vi "Dashboard Main.vi"() -> ()   [LabVIEW 2012]
uses:
  <vilib>/Utility/sysdir.llb/System Directory Type.ctl
  <vilib>/event_ctls.llb/eventvkey.ctl
  <vilib>/Utility/config.llb/Read Key (String).vi
  <vilib>/Utility/config.llb/Read Key (I32).vi
  <vilib>/Utility/config.llb/Write Key (String).vi
  <vilib>/Utility/config.llb/Write Key (I32).vi
  <vilib>/Utility/config.llb/NI_LVConfig.lvlib
panel:
  out "PitchMin":dbl
  out "PitchMax":dbl
  in  "Auto Align OFF":bool
  in  "Auto Pitch OFF":bool
  in  "Enabled Overlay":T1
  out "Status":T2(ring)
  out "Pitch MotorSlide":dbl(slide) scale=-1.0..1.0 scale format="%#_2e"
  out "Pitch MotorChart":dbl(graph)
  out "Shooter MotorSlide":dbl(slide) scale=-1.0..1.0 scale format="%#_2e"
  out "Shooter MotorChart":dbl(graph)
  out "Battery Value":dbl(slide) scale=0.0..14.0 scale format="%#_2e"
  out "Battery":sgl(graph)
  out "Robot IP":string
  out "JS1 Z":dbl(slide) scale=-1.0..1.0 scale format="%#_2e"
  out "JS2 Z":dbl(slide) scale=-1.0..1.0 scale format="%#_2e"
  out "Joystick 1":cluster{"X":dbl, "Y":dbl}[](graph)
  out "Joystick 2":cluster{"X":dbl, "Y":dbl}[](graph)
  out "JS Buttons 1":T3
  out "JS Buttons 2":T3
  out "MotorSlide4":dbl(slide) scale=-1.0..1.0 scale format="%#_2e"
  out "MotorChart4":dbl(graph)
  out "MotorSlide3":dbl(slide) scale=-1.0..1.0 scale format="%#_2e"
  out "MotorSlide2":dbl(slide) scale=-1.0..1.0 scale format="%#_2e"
  out "MotorChart3":dbl(graph)
  out "MotorChart2":dbl(graph)
  out "MotorSlide1":dbl(slide) scale=-1.0..1.0 scale format="%#_2e"
  out "MotorChart1":dbl(graph)
  out "Buttons 1":cluster{"1":bool, "2":bool, "3":bool}
  out "Kinect 1":cluster{"X":dbl, "Y":dbl, "Z":dbl} {"X" scale=1.0..-1.0; "Y" scale=1.0..-1.0; "Z" scale=1.0..-1.0}
  out "Buttons 2":cluster{"1":bool, "2":bool, "3":bool}
  out "Kinect 2":cluster{"X":dbl, "Y":dbl, "Z":dbl} {"X" scale=1.0..-1.0; "Y" scale=1.0..-1.0; "Z" scale=1.0..-1.0}
  out "Version":string
  out "Skeleton Picture":picture
  out "Players":i8
  out "Image Error":errorcluster
  in  "Camera Settings":T4={"Frate Rate"=15, "Compression"=49, "Size"=1} {"Frate Rate" scale=1.0..30.0; "Size" items=["640x480", "320x240", "160x120"]}
  out "Camera IP":string
  in  "Dashboard Tab":T5(tab)
  in  "Mark PitchF":bool
  in  "Current Pitch":dbl
  in  "Pitch Firing":dbl
  in  "Pitch Loading":dbl
  in  "AutoTargetPitch":dbl
  out "Invert Drive":bool
  out "Fine Control Mode":bool
  out "KickerOut":dbl
  out "Angel Eye":bool
  out "Auto Align":bool
  in  "AutoTargetRotation":dbl
  out "Mode":T6(ring)=enum."Auto Disabled"
  out "# of records":i64
  in  "Mark":bool
  out "Distance":string
  out "Full Array":dbl[][](array[numeric])
  out "SelectedGoalSubarray":dbl[](array[numeric])
  in  "Slider":dbl(slide) scale=0.0..100.0 scale format="%#_3g"
  in  "On/Off":bool caption="Solenoid"
  in  "Test Name":u16(ring) items=["Select the test to run...", "Example Test", "-------------------------------", "List of tests is built in robot code.", "Replace with your own automated tests."]
  in  "Test Tree":string(tree)
  in  "Motor":cluster{"Value":dbl, "Enable":bool} {"Value" scale=-1.0..1.0 scale format="%#_3g"}
  out "Progress":T7 {"Test Progress" scale=0.0..100.0}
  in  "Rev/Fwd":cluster{"Forward":bool, "Reverse":bool}
  in  "Ring":u16(ring) items=["Auto", "Fixed indoor", "Fixed outdoor 1", "Fixed outdoor 2", "Fixed fluorescent 1", "Fixed fluorescent 2", "Hold current"]
  in  "Listbox":i32(listbox)
  in  "Viewer":enum32{"Camera Image", "Variables"}(tab)
  out "Mbps":dbl format="%#.1g"
  in  "Enable":bool
  in  "DB Camera Config":bool
  out "Mbps":bool
  out "fps":dbl format="%#.1g"
  out "Image Error Message":string="Timeout in Camera Communications"
  out "Camera Image":T8(plugin-control)
  out "Tree":string(tree)
  out "Boolean 7":bool
  out "Boolean 6":bool
  out "Boolean 5":bool
  out "Boolean 4":bool
  out "Boolean 3":bool
  out "Boolean 2":bool
  out "Boolean":bool
  # "Drive & Motors"
  # "Rear Left"
  # "Rear Right"
  # "Front Left"
  # "Front Right"
  # "Shooter"
  # "Pitch Control"
  # "Robot IP:"
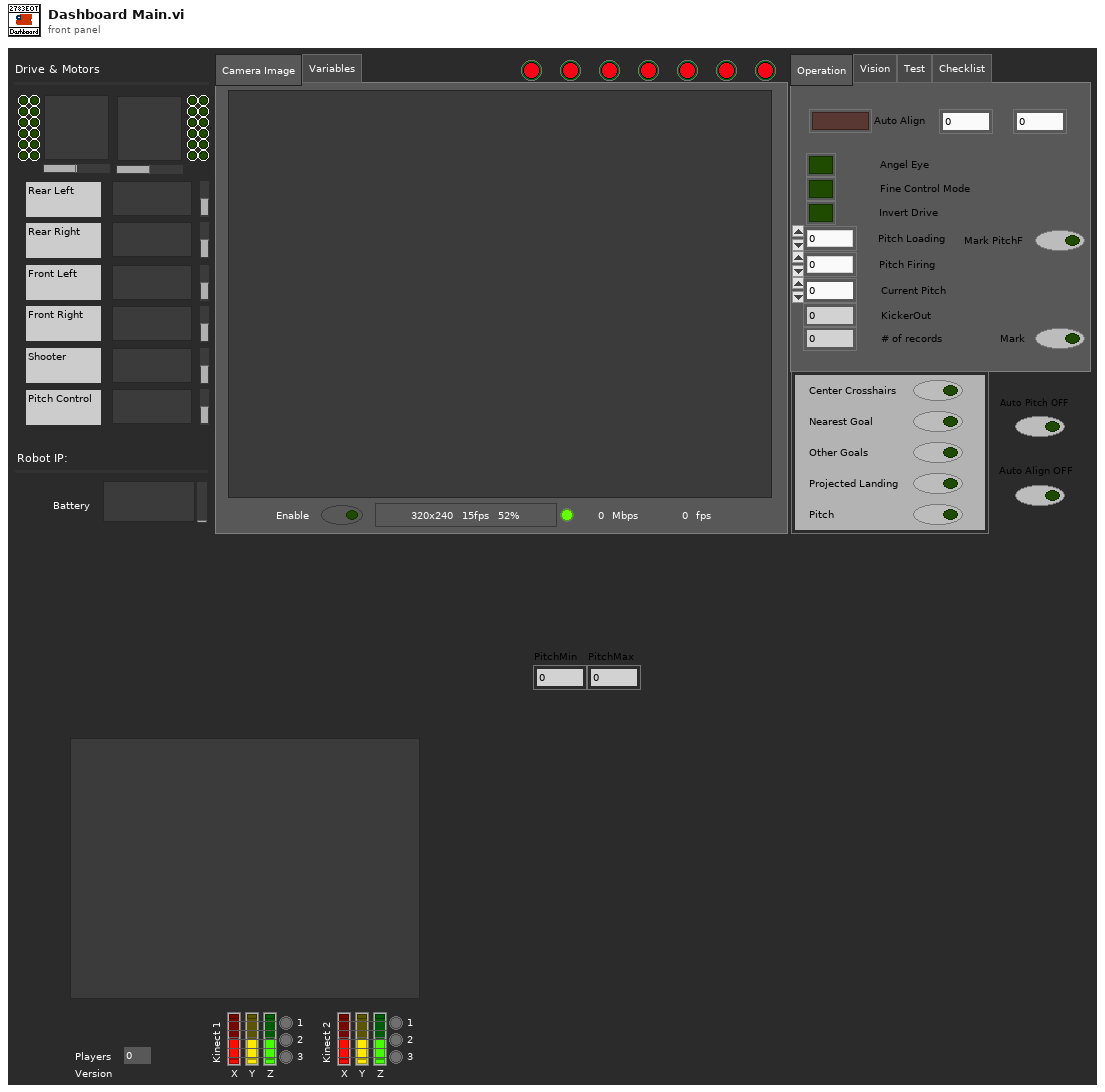
[diagram p1: front panel]
types:
  T1 = cluster{"Center Crosshairs":bool, "Nearest Goal":bool, "Other Goals":bool, "Projected Landing":bool, "Pitch":bool}
  T2 = enum8{"Disconnected", "E-Stop", "Disabled", "Enabled"}
  T3 = cluster{bool, bool, bool, bool, bool, bool, bool, bool, bool, bool, bool, bool}
  T4 = cluster{"Frate Rate":i32, "Compression":i32, "Size":u16}
  T5 = enum32{"Operation", "Vision", "Test", "Checklist"}
  T6 = enum8{"Tele-Op Disabled", "Tele-Op Enabled", "Auto Disabled", "Auto Enabled", "Test Disabled", "Test Enabled", ""}
  T7 = cluster{"Test Progress":u8, "Test Progress Text":string}
  T8 = typedef "IMAQ Image.ctl" = refnum<image>
  T9 = cluster{"Time":string, "Step":string, "Description":string}
  T10 = enum16{"open", "replace", "create", "open or create", "replace or create", "replace or create with confirmation"}
  T11 = cluster{"Joystick 1":cluster{"X":dbl, "Y":dbl}[], "JS Buttons 1":cluster{bool, bool, bool, bool, bool, bool, bool, bool, bool, bool, bool, bool}, "Joystick 2":cluster{"X":dbl, "Y":dbl}[], "JS Buttons 2":cluster{bool, bool, bool, bool, bool, bool, bool, bool, bool, bool, bool, bool}, "AutoTargetRotation":dbl, "AutoTargetPitch":dbl, "Fine Control Mode":bool, "Auto Align":bool, "Current Pitch":dbl, "Full Array":dbl[][], "SelectedGoalSubarray":dbl[], "Distance":string}
  T12 = typedef "System Directory Type.ctl" = i32
  T13 = typedef "Image Type" = u32
  T14 = typedef "AviRefnum.ctl" = refnum<k1>
  T15 = typedef "LVBoundsTypeDef.ctl" = cluster{"Width":u32, "Height":u32}
  T16 = typedef "SkeletonTrackState.ctl" = enum32{"NotTracked", "PositionOnly", "Tracked"}
  T17 = cluster{"TrackingState":u8[], "Position":cluster{"x":sgl, "y":sgl, "z":sgl}, cluster{"x":sgl, "y":sgl, "z":sgl, sgl}[], "TrackState":T16}
  T18 = cluster{cluster{"ScaledToPercentRange":dbl, "ScaledToPercentRange":dbl, "ScaledToPercentRange":dbl}, cluster{bool, bool, bool}}[]
  T19 = cluster{cluster{"ScaledToPercentRange":dbl, "ScaledToPercentRange":dbl, "ScaledToPercentRange":dbl}, cluster{bool, bool, bool}}
  T20 = cluster{"ScaledToPercentRange":dbl, "ScaledToPercentRange":dbl, "ScaledToPercentRange":dbl}
  T21 = typedef "LVRectTypeDef.ctl" = cluster{"Left":i16, "Top":i16, "Right":i16, "Bottom":i16}
  T22 = cluster{"PitchMin":dbl, "PitchMax":dbl, "Pitch Firing":dbl, "Pitch Loading":dbl, "Current Pitch":dbl}
  T23 = cluster{"Competition mode":bool, "Robot Link":bool, "Autonomous":bool, "Enabled":bool, "E-Stop":bool, "Simulated":bool, "TestMode":bool, "Docked Window":bool}
  T24 = cluster{"Boolean Array[0]":bool, "Boolean Array[1]":bool, "Boolean Array[2]":bool, "Boolean Array[3]":bool, "Boolean Array[4]":bool, "Boolean Array[5]":bool, "Boolean Array[6]":bool, "Boolean Array[7]":bool, "Boolean Array[8]":bool, "Boolean Array[9]":bool, "Boolean Array[10]":bool, "Boolean Array[11]":bool}
  T25 = typedef "NI_LVConfig.lvlib/Config Data RefNum.ctl" = refnum<k1>
  T26 = typedef "eventvkey.ctl" = enum16{"ASCII", "Enter", "Return", "Shift", "Ctrl", "Alt", "Cmd", "Opt", "Caps", "NumLock", "Clear", "Break", "Up", "Down", "Left", "Right", "Insert", "Delete", "Home", "End", "PageUp", "PageDown", "Escape", "Help", "Pause", "ScrollLock", "F1", "F2", "F3", "F4", "F5", "F6", "F7", "F8", "F9", "F10", "F11", "F12", "F13", "F14", "F15", "F16", "F17", "F18", "F19", "F20", "F21", "F22", "F23", "F24", "Play", "VolumeUp", "VolumeDown", "Mute", "Two Byte Char"}
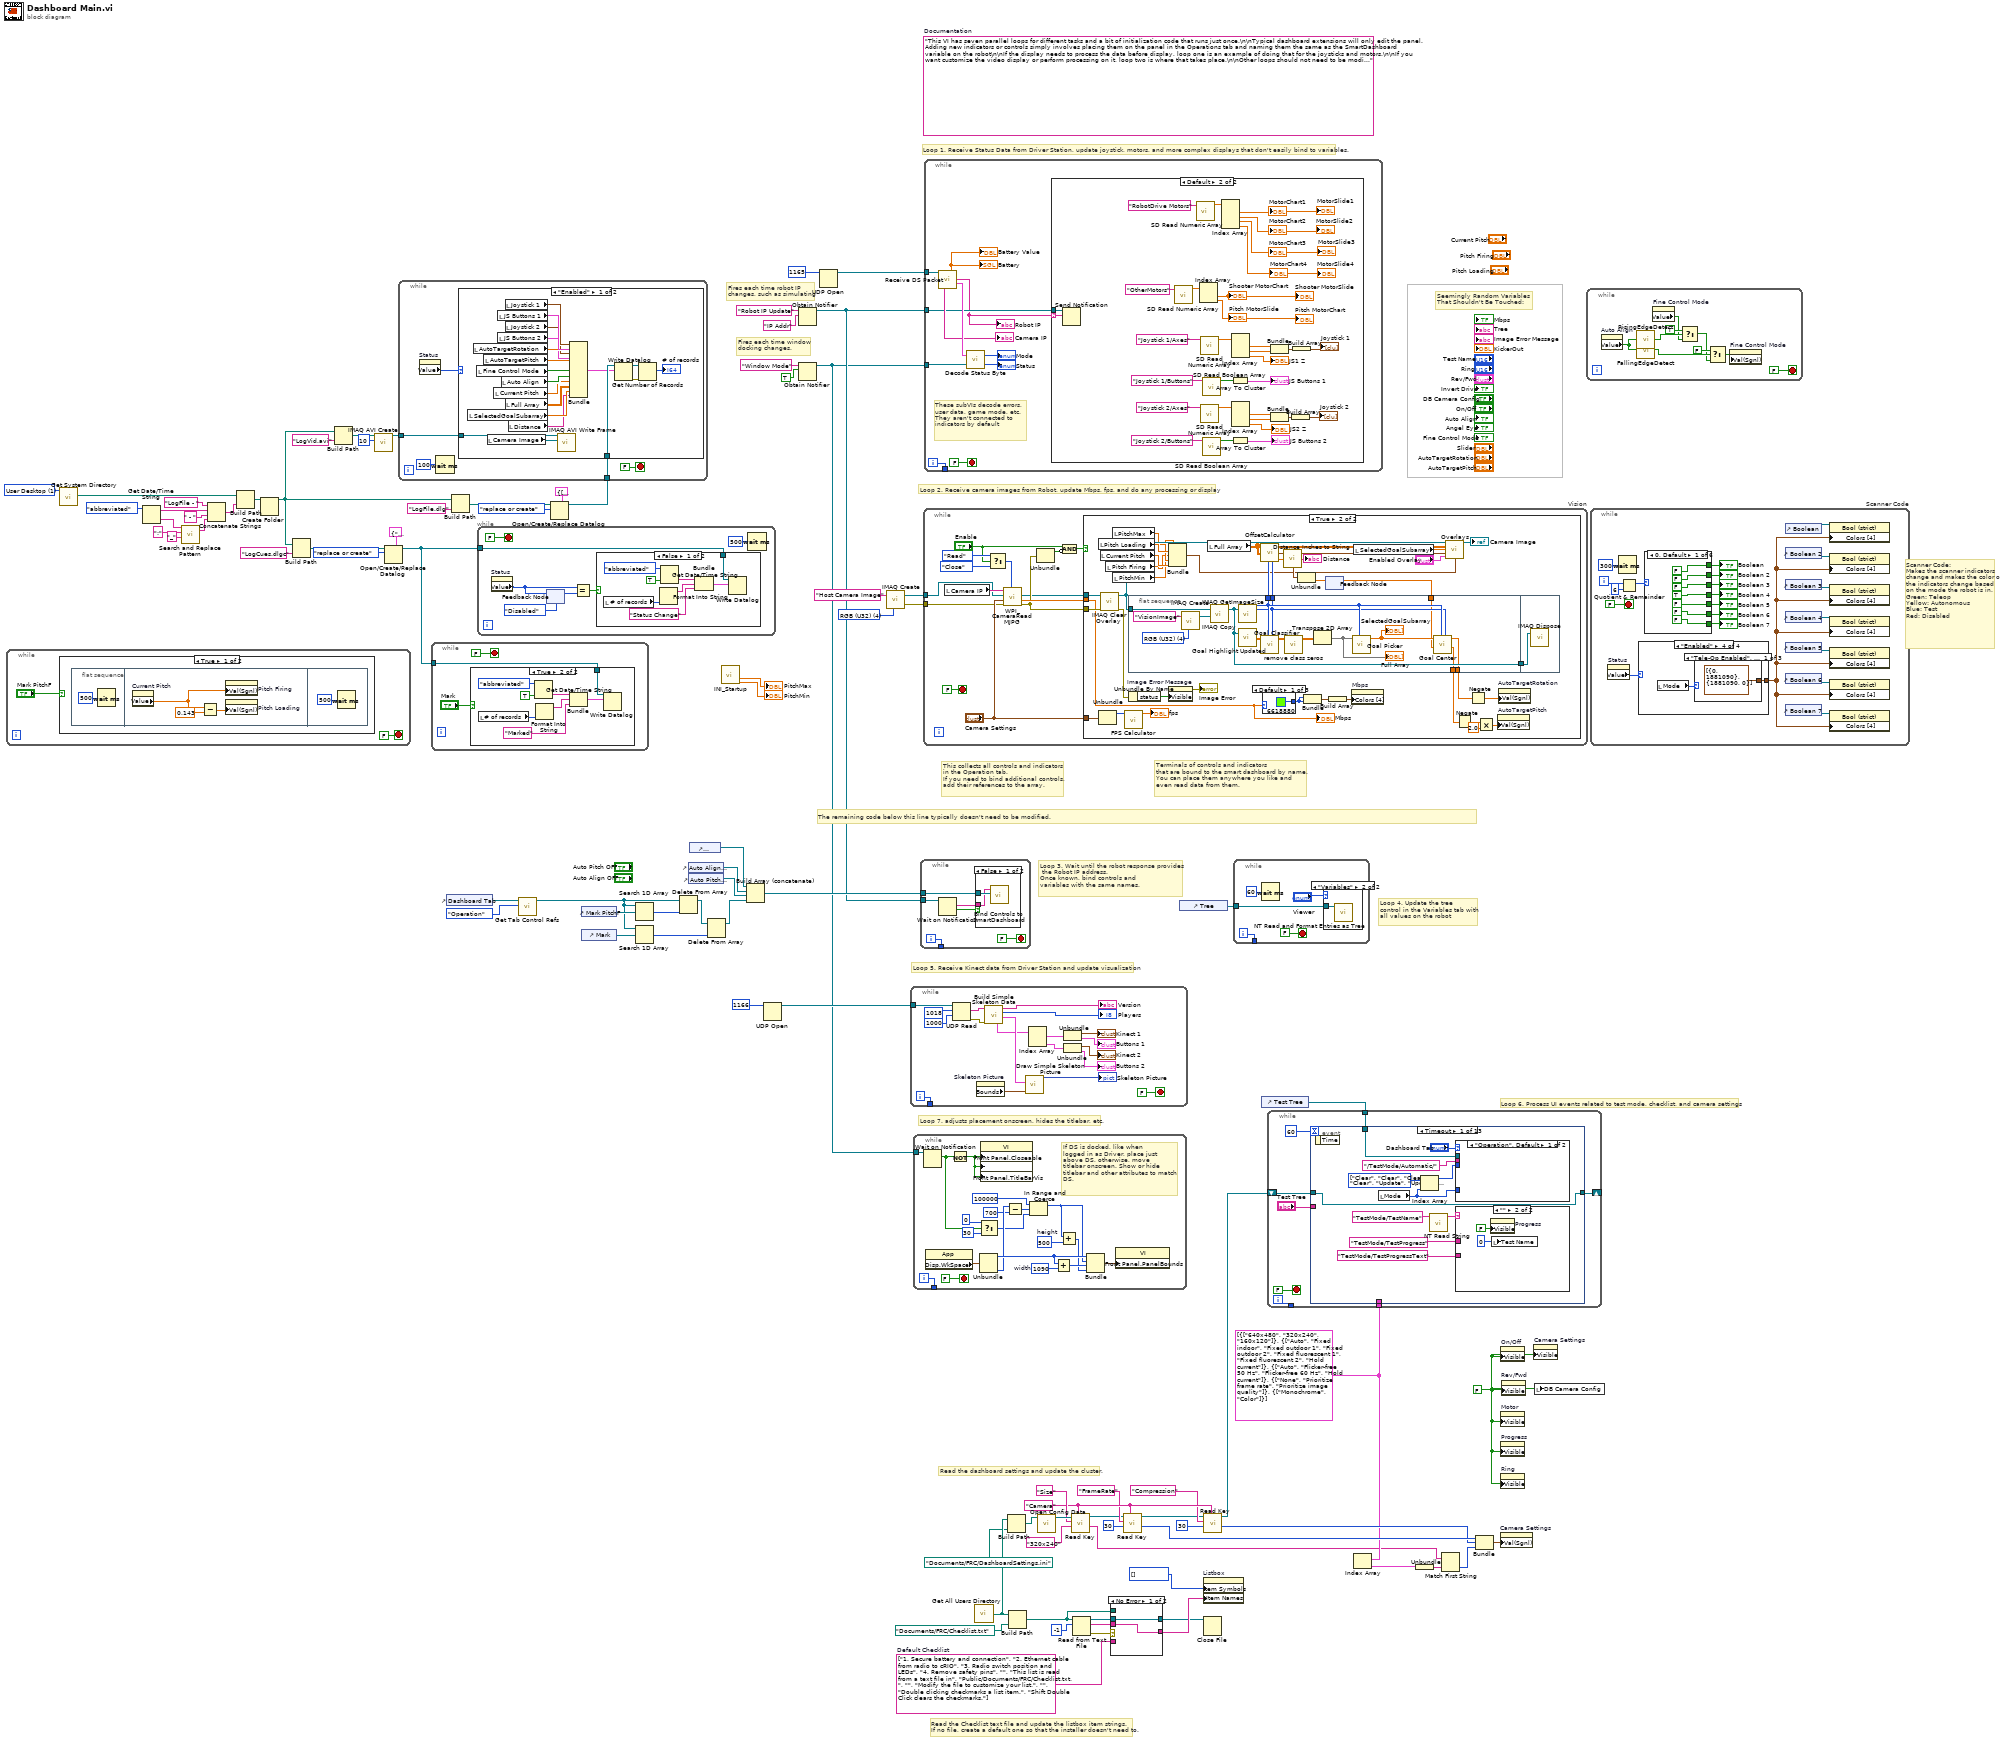
[diagram p0: block diagram]
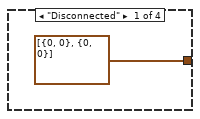
[diagram p6: hidden frame]
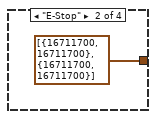
[diagram p7: hidden frame]
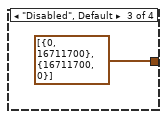
[diagram p8: hidden frame]
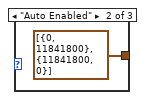
[diagram p9: hidden frame]
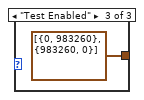
[diagram p10: hidden frame]
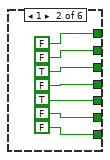
[diagram p11: hidden frame]
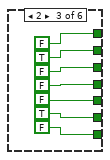
[diagram p12: hidden frame]
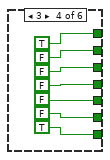
[diagram p13: hidden frame]
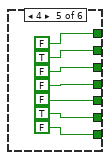
[diagram p14: hidden frame]
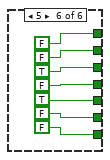
[diagram p15: hidden frame]
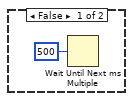
[diagram p17: hidden frame]
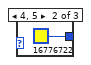
[diagram p18: hidden frame]
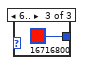
[diagram p19: hidden frame]
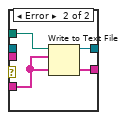
[diagram p20: hidden frame]
diagram:
  w36 = T12 1 items=["User Home"=0, "User Desktop"=1, "User Documents"=2, "User Application Data"=3, "User Preferences"=4, "User Temporary"=5, "Public Documents"=6, "Public Application Data"=7, "Public Preferences"=8, "Public Cache"=13, "System Core Libraries"=9, "System Installed Libraries"=10, "Application Files"=11, "Boot Volume Root"=12] ("system directory type")
  w62 = "Camera"
  w54 = cluster{string[]}[] [{["640x480", "320x240", "160x120"]}, {["Auto", "Fixed indoor", "Fixed outdoor 1", "Fixed outdoor 2", "Fixed fluorescent 1", "Fixed fluorescent 2", "Hold current"]}, {["Auto", "Flicker-free 50 Hz", "Flicker-free 60 Hz", "Hold current"]}, {["None", "Prioritize frame rate", "Prioritize image quality"]}, {["Monochrome", "Color"]}]
  w70 = string[] ["1. Secure battery and connection", "2. Ethernet cable from radio to cRIO", "3. Radio switch position and LEDs", "4. Remove safety pins", "", "This list is read from a text file in", "Public/Documents/FRC/Checklist.txt.", "", "Modify the file to customize your list.", "", "Double clicking checkmarks a list item.", "Shift Double Click clears the checkmarks."]  # Default Checklist
  w68 = FALSE ("Visible")
  (unwired) "This VI has seven parallel loops for different tasks and a bit of initialization code that runs just once.\n\nTypical dashboard extensions will only edit the panel. Adding new indicators or controls simply involves placing them on the panel in the Operations tab and naming them the same as the SmartDashboard variable on the robot\n\nIf the display needs to process the data before display, loop one is an example of doing that for the joysticks and motors.\n\nIf you want customize the video display or perform processing on it, loop two is where that takes place.\n\nOther loops should not need to be modified. They are pretty standard, and document the task they perform."  # Documentation
  w88 = T13 4 items=["Grayscale (U8)", "Grayscale (I16)", "Grayscale (SGL)", "Complex (CSG)", "RGB (U32)", "HSL (U32)", "RGB (U64)"] ("Image Type")
  # "Scanner Code:\nMakes the scanner indicators change and makes the color of the indicators change based on the mode the robot is in.\nGreen: Teleop\nYellow: Autonomous\nBlue: Test\nRed: Disabled"
  # "Seemingly Random Variables That Shouldn't Be Touched:"
  # "Fires each time robot IP\nchanges, such as simulating"
  # "Fires each time window\ndocking changes."
  # "Read the Checklist text file and update the listbox item strings.\nIf no file, create a default one so that the installer doesn't need to."
  # "This collects all controls and indicators\nin the Operation tab.\nIf you need to bind additional controls,\nadd their references to the array."
  # "The remaining code below this line typically doesn't need to be modified."
  # "Loop 6. Process UI events related to test mode, checklist, and camera settings"
  # "Read the dashboard settings and update the cluster."
  # "Terminals of controls and indicators\nthat are bound to the smart dashboard by name.\nYou can place them anywhere you like and\neven read data from them."
  # "Loop 4. Update the tree\ncontrol in the Variables tab with\nall values on the robot"
  # "Loop 3. Wait until the robot response provides\n the Robot IP address.\nOnce known, bind controls and\nvariables with the same names."
  # "Loop 5. Receive Kinect data from Driver Station and update visualization"
  # "Loop 7. adjusts placement onscreen, hides the titlebar, etc."
  # "Loop 1. Receive Status Data from Driver Station, update joystick, motors, and more complex displays that don't easily bind to variables."
  # "Loop 2. Receive camera images from Robot, update Mbps, fps, and do any processing or display"
  n1 = while {
    stop <- FALSE stop-if-true
    n2 = case shown="True" "Mark PitchF" {
      frame True {
        n3 = flat-sequence {
          frame #0 {
            n4 = Wait (ms)(milliseconds to wait=u32 500) -> ()  [unwired: 1 out]
          }
          frame #1 {
            n5 = property on="Current Pitch" class="DigNum (strict)"() -> ("Value"=w96:dbl)  [unwired: 2 in, 2 out]
            n6 = Subtract(x=w96, y=0.143) -> (x-y=w97:dbl)
            n7 = property on="Pitch Firing" class="DigNum (strict)"("Val(Sgnl)"=w96) -> ()  [unwired: 2 in, 2 out]
            n8 = property on="Pitch Loading" class="DigNum (strict)"("Val(Sgnl)"=w97) -> ()  [unwired: 2 in, 2 out]
          }
          frame #2 {
            n9 = Wait (ms)(milliseconds to wait=u32 500) -> ()  [unwired: 1 out]
          }
        }
      }
      frame False {
      }
    }
  }
  n10 = call <vilib>:"Get System Directory.vi"("system directory type"=w36) -> ("system directory"=w25:path)  [unwired: 10 in]
  n11 = Get Date/Time String(date format (0)=enum16{"short", "long", "abbreviated"}."abbreviated") -> (date string=w23:string, time string=w17:string)  [unwired: 2 in]
  n12 = call <vilib>:"Search and Replace Pattern.vi"("string"=w17, "regular expression (\"\")"=":" ("search string/char (-)"), "replace string (\"\")"="_" ("replace string (\"\")")) -> ("result string"=w20:string)  [unwired: 2 in, 1 out]
  n13 = Concatenate Strings("LogFile - " ("string"), w23, " - " ("string"), w20) -> (w21:string)
  n14 = Build Path(base path=w25, name or relative path=w21) -> (appended path=w27:path)
  n15 = Create Folder(path (use dialog)=w27) -> (created path=w12:path)  [unwired: 2 in, 2 out]
  n16 = Build Path(base path=w12, name or relative path="LogCues.dlgc") -> (appended path=w10:path)
  n17 = Build Path(base path=w12, name or relative path="LogVid.avi") -> (appended path=w29:path)
  n18 = call "IMAQ AVI Create"("Frames Per Second"=u32 10, "AVI Path"=w29) -> ("Avi Refnum"=w28:T14)  [unwired: 8 in, 1 out]
  n19 = Open/Create/Replace Datalog(5:T9 {"Time"="", "Step"="", "Description"=""}, 10:T10."replace or create" ("operation (0:open)"), 11:w10) -> (3:w8:refnum<k1>)  [unwired: 3 in, 2 out]
  n20 = while {
    tunnel: w8 -> [w100]
    stop <- FALSE stop-if-true
    n21 = case shown="True" "Mark" {
      tunnel: w100 -> [_ w105]
      frame False {
      }
      frame True {
        n22 = local read "# of records"() -> (w102:i64)
        n23 = Get Date/Time String(date format (0)=enum16{"short", "long", "abbreviated"}."abbreviated", want seconds? (F)=TRUE) -> (time string=w109:string)  [unwired: 1 in, 1 out]
        n24 = Format Into String(w102) -> (resulting string=w103:string)  [unwired: 3 in, 1 out]
        n25 = Bundle("time string"=w109, w103, "Marked") -> (w104:cluster{"time string":string, string, string})  [unwired: 1 in]
        n26 = Write Datalog(6:w104, 7:w105) -> ()  [unwired: 1 in, 2 out]
      }
    }
  }
  n27 = control-ref of="Dashboard Tab"() -> (w84:refnum<vi>)
  n28 = Build Path(base path=w12, name or relative path="LogFile.dlg") -> (appended path=w35:path)
  n29 = while {
    tunnel: w8 -> [w114]
    stop <- FALSE stop-if-true
    n30 = property on="Status" class="Enum (strict)"() -> ("Value"=w111:T2)  [unwired: 2 in, 2 out]
    n31 = feedback-in #1(w111) -> ()
    n32 = feedback #1(T2."Disabled" ("Status")) -> (w112:T2)
    n33 = Equal?(x=w111, y=w112) -> (x = y?=w115:bool)
    n34 = case shown="False" w115 {
      tunnel: w114 -> [w119 _]
      frame False {
        n35 = local read "# of records"() -> (w117:i64)
        n36 = Format Into String(w117) -> (resulting string=w118:string)  [unwired: 3 in, 1 out]
        n37 = Get Date/Time String(date format (0)=enum16{"short", "long", "abbreviated"}."abbreviated", want seconds? (F)=TRUE) -> (time string=w124:string)  [unwired: 1 in, 1 out]
        n38 = Bundle("time string"=w124, w118, "Status Change") -> (w120:cluster{"time string":string, string, string})  [unwired: 1 in]
        n39 = Write Datalog(6:w120, 7:w119) -> ()  [unwired: 1 in, 2 out]
      }
      frame True {
      }
    }
    n40 = Wait (ms)(milliseconds to wait=u32 500) -> ()  [unwired: 1 out]
  }
  n41 = call <vilib>:"Get Tab Control Refs.vi"("Page Index"=enum32{"Operation", "Test"}."Operation" ("Dashboard Tab"), "TabControl in"=w84) -> ("ControlsOnPage"=w1:refnum<vi>[])  [unwired: 9 in]
  n42 = Open/Create/Replace Datalog(5:T11 {"Joystick 1"=[], "JS Buttons 1"={FALSE, FALSE, FALSE, FALSE, FALSE, FALSE, FALSE, FALSE, FALSE, FALSE, FALSE, FALSE}, "Joystick 2"=[], "JS Buttons 2"={FALSE, FALSE, FALSE, FALSE, FALSE, FALSE, FALSE, FALSE, FALSE, FALSE, FALSE, FALSE}, "AutoTargetRotation"=0.0, "AutoTargetPitch"=0.0, "Fine Control Mode"=FALSE, "Auto Align"=FALSE, "Current Pitch"=0.0, "Full Array"=[], "SelectedGoalSubarray"=[], "Distance"=""} ("output cluster"), 10:T10."replace or create" ("operation (0:open)"), 11:w35) -> (3:w33:refnum<k1>)  [unwired: 3 in, 2 out]
  n43 = while {
    tunnel: w33 -> [w129]
    tunnel: w28 -> [w126]
    stop <- FALSE stop-if-true
    n44 = property on="Status" class="Enum (strict)"() -> ("Value"=w125:T2)  [unwired: 2 in, 2 out]
    n45 = Wait (ms)(milliseconds to wait=u32 100) -> ()  [unwired: 1 out]
    n46 = case shown="\"Enabled\"" w125 {
      tunnel: w129 -> [w148 _]
      tunnel: w126 -> [w133 _]
      frame "Enabled" {
        n47 = local read "SelectedGoalSubarray"() -> (w137:dbl[])
        n48 = local read "AutoTargetRotation"() -> (w143:dbl)
        n49 = local read "Fine Control Mode"() -> (w141:bool)
        n50 = local read "AutoTargetPitch"() -> (w142:dbl)
        n51 = local read "Camera Image"() -> (w134:T8)
        n52 = local read "Current Pitch"() -> (w139:dbl)
        n53 = local read "JS Buttons 1"() -> (w146:T3)
        n54 = local read "JS Buttons 2"() -> (w144:T3)
        n55 = local read "Auto Align"() -> (w140:bool)
        n56 = local read "Joystick 1"() -> (w147:cluster{"X":dbl, "Y":dbl}[])
        n57 = local read "Joystick 2"() -> (w145:cluster{"X":dbl, "Y":dbl}[])
        n58 = local read "Full Array"() -> (w138:dbl[][])
        n59 = local read "Distance"() -> (w135:string)
        n60 = call "IMAQ AVI Write Frame"("Image"=w134, "Avi Refnum"=w133) -> ()  [unwired: 8 in, 2 out]
        n61 = Bundle("Joystick 1"=w147, "JS Buttons 1"=w146, "Joystick 2"=w145, "JS Buttons 2"=w144, "AutoTargetRotation"=w143, "AutoTargetPitch"=w142, "Fine Control Mode"=w141, "Auto Align"=w140, "Current Pitch"=w139, "Full Array"=w138, "SelectedGoalSubarray"=w137, "Distance"=w135) -> (w136:T11)  [unwired: 1 in]
        n62 = Write Datalog(6:w136, 7:w148) -> (0:w131:errorcluster, 3:w132:refnum<k1>)  [unwired: 1 in]
        n63 = Get Number of Records(4:w131, 7:w132) -> (2:→"# of records":i64)  [unwired: 2 out]
      }
      frame "Disabled", Default {
      }
    }
  }
  n64 = control-ref of="Mark PitchF"() -> (w6:refnum<vi>)
  n65 = control-ref of="Mark"() -> (w7:refnum<vi>)
  n66 = Search 1D Array(1D array=w1, element=w6) -> (index of element=w5:i32)  [unwired: 1 in]
  n67 = Search 1D Array(1D array=w1, element=w7) -> (index of element=w4:i32)  [unwired: 1 in]
  n68 = Delete From Array(array=w1, index=w5) -> (array with subset deleted=w3:refnum<vi>[])  [unwired: 1 in, 1 out]
  n69 = control-ref of="Auto Align OFF"() -> (w39:refnum<vi>)
  n70 = control-ref of="Auto Pitch OFF"() -> (w38:refnum<vi>)
  n71 = control-ref of="AutoTargetPitch"() -> (w37:refnum<vi>)
  n72 = Delete From Array(array=w3, index=w4) -> (array with subset deleted=w2:refnum<vi>[])  [unwired: 1 in, 1 out]
  n73 = call "INI_Startup.vi"() -> ("PitchMin"=→"PitchMin":dbl, "PitchMax"=→"PitchMax":dbl)  [unwired: 4 in, 2 out]
  n74 = Build Array (concatenate)(w37, w39, w38, w2) -> (w91:refnum<vi>[])
  n75 = UDP Open(11:u16 1166 ("port")) -> (port=w85:refnum<k16>)  [unwired: 2 in, 4 out]
  n76 = Obtain Notifier(name (unnamed)="Robot IP Update", notification data type="IP Addr" ("name (unnamed)")) -> (notifier out=w81:refnum<notifier>)  [unwired: 2 in, 2 out]
  n77 = Obtain Notifier(name (unnamed)="Window Mode", notification data type=TRUE) -> (notifier out=w74:refnum<notifier>)  [unwired: 2 in, 2 out]
  n78 = UDP Open(11:u16 1165 ("port")) -> (port=w89:refnum<k16>)  [unwired: 2 in, 4 out]
  n79 = call "IMAQ Create"("Image Name"="Host Camera Image", "Image Type"=w88) -> ("New Image"=w41:T8, "error out"=w40:errorcluster)  [unwired: 2 in, 1 out]
  n80 = while {
    tunnel: w85 -> [w165]
    tunnel: [w150] -> _
    i -> [w150]
    stop <- FALSE stop-if-true
    n81 = UDP Read(connection ID=w165, max size (548)=1018 ("bytes to read"), timeout ms (25000)=1000) -> (data out=w159:string, error out=w149:errorcluster)  [unwired: 1 in, 3 out]
    n82 = property on="Skeleton Picture" class="Pict"() -> ("Bounds"=w161:T15)  [unwired: 2 in, 2 out]
    n83 = call "Build Simple Skeleton Data.vi"("error in (no error)"=w149, "data in"=w159) -> ("Skeleton Data"=w160:T17, "NumPlayers"=→"Players":i8, "Version String"=→"Version":string, "Simple Joystick Info"=w157:T18)  [unwired: 5 in, 1 out]
    n84 = call "Draw Simple Skeleton Picture.vi"("Bounds"=w161, "Simple Skeleton"=w160) -> ("new picture out"=→"Skeleton Picture":picture)  [unwired: 9 in]
    n85 = Index Array(array=w157) -> (element #1=w156:T19, element #2=w155:T19)  [unwired: 2 in]
    n86 = Unbundle(w156) -> (→"Kinect 1":T20, →"Buttons 1":cluster{bool, bool, bool})
    n87 = Unbundle(w155) -> (→"Kinect 2":T20, →"Buttons 2":cluster{bool, bool, bool})
  }
  n88 = while {
    tunnel: w74 -> [w186]
    tunnel: [w185] -> _
    i -> [w185]
    stop <- FALSE stop-if-true
    w177 = 1090  # width
    w180 = 500  # height
    # "If DS is docked, like when\nlogged in as Driver, place just\nabove DS, otherwise, move\ntitlebar onscreen. Show or hide\ntitlebar and other attributes to match\nDS."
    n89 = Wait on Notification(notifier=w186) -> (notification=w172:bool)  [unwired: 3 in, 3 out]
    n90 = property class="App"() -> ("Disp.WkSpace"=w183:T21)  [unwired: 2 in, 2 out]
    n91 = Not(x=w172) -> (.not. x?=w168:bool)
    n92 = Unbundle(w183) -> ("Left"=w181:i16, "Bottom"=w178:i16)  [unwired: 2 out]
    n93 = Select(t=0, s=w172, f=30) -> (s? t:f=w171:i32)
    n94 = property class="VI"("Front Panel.Closeable"=w168, "Front Panel.Minimizeable"=w168, "Front Panel.TitleBarVis"=w168) -> ()  [unwired: 2 in, 2 out]
    n95 = Subtract(x=w178, y=700) -> (x-y=w175:i32)
    n96 = In Range and Coerce(upper limit=100000, x=w175, lower limit=w171) -> (coerced(x)=w169:i32)  [unwired: 1 out]
    n97 = Add(x=w181, y=w177) -> (x+y=w182:i32)
    n98 = Add(x=w169, y=w180) -> (x+y=w179:i32)
    n99 = Bundle("Left"=w181, w169, w182, w179) -> (w184:cluster{"Left":i16, i32, i32, i32})  [unwired: 1 out]
    n100 = property class="VI"("Front Panel.PanelBounds"=w184) -> ()  [unwired: 2 in, 2 out]
  }
  n101 = while {
    tunnel: w91 -> [w193]
    tunnel: w81 -> [w190]
    tunnel: [w188] -> _
    i -> [w188]
    stop <- FALSE stop-if-true
    n102 = Wait on Notification(notifier=w190) -> (notification=w189:string, timed out?=w191:bool)  [unwired: 3 in, 2 out]
    n103 = case shown="False" w191 {
      tunnel: w193 -> [w195 _]
      tunnel: w189 -> [w194 _]
      frame False {
        n104 = call <vilib>:"Bind Controls to SmartDashboard.vi"("Bound Control Refs"=w195, "Server IP Address"=w194) -> ()  [unwired: 10 in]
      }
      frame True {
      }
    }
  }
  n105 = while "Vision" {
    tunnel: w40 -> [w199]
    tunnel: w41 -> [w197]
    stop <- FALSE stop-if-true
    n106 = local read "Camera IP"() -> (w208:string)
    n107 = Select(t=enum16{"Read", "Reopen", "Close"}."Read" ("Operation"), s="Enable", f=enum16{"Read", "Reopen", "Close"}."Close" ("Operation")) -> (s? t:f=w203:enum16{"Read", "Reopen", "Close"})
    n108 = call <vilib>:"WPI_CameraRead MJPG.vi"("Operation"=w203, "error in"=w199, "Camera Settings"="Camera Settings", "Image"=w197, "address"=w208) -> ("error out"=w198:errorcluster, "Bandwidth (kbps)"=w206:dbl, "Image Out"=w196:T8)  [unwired: 4 in]
    n109 = Unbundle(w198) -> ("status"=w201:bool)  [unwired: 2 out]
    n110 = Compound Arithmetic op=AND("Enable", invert w201) -> (w200:bool)
    n111 = case shown="True" w200 {
      tunnel: "Camera Settings" -> [_ w242]
      tunnel: w206 -> [_ w226]
      tunnel: w198 -> [_ w239]
      tunnel: w196 -> [_ w238]
      frame False {
        n112 = Wait Until Next ms Multiple(millisecond multiple=u32 500) -> ()  [unwired: 1 out]
      }
      frame True {
        n113 = local read "Pitch Loading"() -> (w215:dbl)
        n114 = Unbundle(w242) -> ("Frate Rate"=w241:i32)  [unwired: 2 out]
        n115 = local read "Current Pitch"() -> (w214:dbl)
        n116 = call "IMAQ Clear Overlay"("error in (no error)"=w239, "Image"=w238) -> ("error out"=w227:errorcluster, "Image Out"=w232:T8)  [unwired: 1 in, 7 out]
        n117 = local read "Pitch Firing"() -> (w213:dbl)
        n118 = local read "PitchMax"() -> (w216:dbl)
        n119 = local read "PitchMin"() -> (w212:dbl)
        n120 = call "FPS Calculator.vi"("Average Count"=w241) -> ("fps"=→"fps":dbl)  [unwired: 10 in]
        n121 = flat-sequence {
          tunnel: w232 -> [w260]
          tunnel: [w257] -> w237
          tunnel: [w252] -> w221
          tunnel: [w251] -> w220
          tunnel: [w250] -> w231
          tunnel: [w249] -> w230
          tunnel: w223 -> [w248]
          tunnel: w237 -> [w263]
          frame #0 {
            w259 = T13 4 items=["Grayscale (U8)", "Grayscale (I16)", "Grayscale (SGL)", "Complex (CSG)", "RGB (U32)", "HSL (U32)", "RGB (U64)", "Grayscale (U16)"] ("Image Type")
            n122 = call "IMAQ Create"("Image Name"="VisionImage", "Image Type"=w259) -> ("New Image"=w261:T8)  [unwired: 3 in, 1 out]
            n123 = call "IMAQ Copy"("Image Dst"=w261, "Image Src"=w260) -> ("Image Dst Out"=w257:T8)  [unwired: 4 in, 1 out]
            n124 = call "IMAQ GetImageSize"("Image"=w257) -> ("Y Resolution"=w249:i32, "X Resolution"=w250:i32)  [unwired: 3 in, 1 out]
            n125 = call "Goal Highlight Updated.vi"("Image In"=w257) -> ("Particle Measurements (Pixels)"=w262:dbl[][])  [unwired: 1 in, 2 out]
            n126 = call "Goal Classifier.vi"("ResolutionY"=w249, "ResolutionX"=w250, "InArray"=w262) -> ("OutArray"=w255:dbl[][])  [unwired: 8 in]
            n127 = call "remove class zeros.vi"("Array In"=w255) -> ("Array Out"=w256:dbl[][])  [unwired: 6 in]
            n128 = Transpose 2D Array(2D array=w256) -> (transposed array=w253:dbl[][])
            "Full Array" <- w253
            n129 = call "Goal Picker.vi"("ResolutionX"=w250, "InArray"=w253) -> ("SelectedGoalSubarray"=w254:dbl[])  [unwired: 8 in]
            "SelectedGoalSubarray" <- w254
            n130 = call "Goal Center.vi"("ResolutionY"=w249, "ResolutionX"=w250, "ProjectedY"=w248, "SelectedGoalSubarray"=w254) -> ("PsuedoJoystickOutPitch"=w251:dbl, "PsuedoJoystickOutRotation"=w252:dbl)  [unwired: 6 in]
          }
          frame #1 {
            n131 = call "IMAQ Dispose"("Image"=w263) -> ()  [unwired: 5 in, 1 out]
          }
        }
        n132 = Unbundle By Name(w227) -> ("status"=w247:bool)
        n133 = property on="Image Error Message" class="Str"("Visible"=w247) -> (error out=→"Image Error":errorcluster)  [unwired: 2 in, 1 out]
        n134 = Bundle("PitchMin"=w212, "PitchMax"=w216, "Pitch Firing"=w213, "Pitch Loading"=w215, "Current Pitch"=w214) -> (w211:T22)  [unwired: 1 in]
        n135 = local read "Full Array"() -> (w229:dbl[][])
        n136 = call "OffsetCalculator.vi"("Array"=w229, "Resolution X"=w231, "Resolution Y"=w230) -> ("ProjectedPosition"=w225:cluster{dbl, dbl}, "Distances (Inches)"=w228:dbl)  [unwired: 5 in]
        n137 = case shown="Default" w226 {
          tunnel: [u32 6618880 ("Color Box") u32 16776722 ("Color Box") u32 16716800 ("Color Box")] -> w244
          frame Default {
          }
          frame 4, 5 {
          }
          frame 6.. {
          }
        }
        n138 = call "Distance Inches to String.vi"("Distance Inches"=w228) -> ("Distance String"=→"Distance":string)
        n139 = Unbundle(w225) -> (w224:dbl)  [unwired: 1 out]
        n140 = Bundle("Color Box"=w244, "Color Box"=w244) -> (w246:cluster{"Color Box":u32, "Color Box":u32})  [unwired: 1 out]
        n141 = feedback #2() -> (w223:dbl)  [unwired: 1 in]
        n142 = feedback-in #2(w224) -> ()
        n143 = Build Array(w246) -> (w245:cluster{"Color Box":u32, "Color Box":u32}[])
        n144 = property on="Mbps" class="Bool (strict)"("Colors [4]"=w245) -> ()  [unwired: 2 in, 2 out]
        n145 = local read "SelectedGoalSubarray"() -> (w234:dbl[])
        n146 = call "Overlays.vi"("Image In"=w232, "FullArray"=w229, "SelectedGoalSubarray"=w234, "ProjectedPosition"=w225, "Enabled Overlay"="Enabled Overlay", "Pitch"=w211) -> ("Image Out"=→"Camera Image":T8)  [unwired: 9 in]
        n147 = Negate(x=w220) -> (-x=w219:dbl)
        n148 = Negate(x=w221) -> (-x=w222:dbl)
        n149 = Multiply(x=w219, y=2.0) -> (x*y=w218:dbl)
        n150 = property on="AutoTargetPitch" class="DigNum (strict)"("Val(Sgnl)"=w218) -> ()  [unwired: 2 in, 2 out]
        n151 = property on="AutoTargetRotation" class="DigNum (strict)"("Val(Sgnl)"=w222) -> ()  [unwired: 2 in, 2 out]
        "Mbps" <- w226
      }
    }
  }
  n152 = while {
    tunnel: w89 -> [w275]
    tunnel: w81 -> [w269]
    tunnel: w74 -> [w273]
    tunnel: [w270] -> _
    i -> [w270]
    stop <- FALSE stop-if-true
    # "These subVIs decode errors, user data, game mode, etc.\nThey aren't connected to indicators by default"
    n153 = call "Receive DS Packet.vi"("Recv Socket"=w275) -> ("Battery"=→"Battery" →"Battery Value":sgl, "Robot IP Address"=w268:string, "Status"=w276:T23, "Camera IP Address"=→"Camera IP":string)  [unwired: 1 in, 10 out]
    "Robot IP" <- w268
    n154 = call "Decode Status Byte.vi"("Window Mode Notifier"=w273, "Status"=w276) -> ("Status"=→"Status":T2, "Mode"=→"Mode":T6)
    n155 = case shown="Default" w268 {
      selector: w268 -> [_ w282]
      tunnel: w269 -> [_ w283]
      frame "0.0.0.0" {
        # "Robot not responding, don't poll the variables"
      }
      frame Default {
        n156 = Send Notification(notification=w282, notifier=w283) -> ()  [unwired: 1 in, 2 out]
        n157 = call <vilib>:"SD Read Numeric Array.vi"("Name"="OtherMotors") -> ("Numeric Array"=w280:dbl[])  [unwired: 8 in, 2 out]
        n158 = call <vilib>:"SD Read Numeric Array.vi"("Name"="RobotDrive Motors") -> ("Numeric Array"=w306:dbl[])  [unwired: 8 in, 2 out]
        n159 = Index Array(array=w280) -> (element #1=→"Shooter MotorChart" →"Shooter MotorSlide":dbl, element #2=→"Pitch MotorSlide" →"Pitch MotorChart":dbl)  [unwired: 2 in]
        n160 = call <vilib>:"SD Read Numeric Array.vi"("Name"="Joystick 1/Axes") -> ("Numeric Array"=w299:dbl[])  [unwired: 8 in, 2 out]
        n161 = call <vilib>:"SD Read Numeric Array.vi"("Name"="Joystick 2/Axes") -> ("Numeric Array"=w293:dbl[])  [unwired: 8 in, 2 out]
        n162 = call <vilib>:"SD Read Boolean Array.vi"("Name"="Joystick 1/Buttons") -> ("Boolean Array"=w301:bool[])  [unwired: 8 in, 2 out]
        n163 = call <vilib>:"SD Read Boolean Array.vi"("Name"="Joystick 2/Buttons") -> ("Boolean Array"=w292:bool[])  [unwired: 8 in, 2 out]
        n164 = Index Array(array=w306) -> (element #1=→"MotorChart1" →"MotorSlide1":dbl, element #2=→"MotorSlide2" →"MotorChart2":dbl, element #3=→"MotorChart3" →"MotorSlide3":dbl, element #4=→"MotorChart4" →"MotorSlide4":dbl)  [unwired: 4 in]
        n165 = Array To Cluster(array=w301) -> (cluster=→"JS Buttons 1":T24)
        n166 = Array To Cluster(array=w292) -> (cluster=→"JS Buttons 2":T24)
        n167 = Index Array(array=w299) -> (element #1=w296:dbl, element #2=w297:dbl, element #3=→"JS1 Z":dbl)  [unwired: 3 in]
        n168 = Index Array(array=w293) -> (element #1=w288:dbl, element #2=w287:dbl, element #3=→"JS2 Z":dbl)  [unwired: 3 in]
        n169 = Bundle("Numeric"=w296, "Numeric"=w297) -> (w295:cluster{"Numeric":dbl, "Numeric":dbl})  [unwired: 1 in]
        n170 = Bundle("Numeric"=w288, "Numeric"=w287) -> (w289:cluster{"Numeric":dbl, "Numeric":dbl})  [unwired: 1 in]
        n171 = Build Array(w289) -> (→"Joystick 2":cluster{"Numeric":dbl, "Numeric":dbl}[])
        n172 = Build Array(w295) -> (→"Joystick 1":cluster{"Numeric":dbl, "Numeric":dbl}[])
      }
    }
  }
  n173 = call "Get All Users Directory.vi"() -> ("All User Path"=w67:path)
  n174 = Build Path(base path=w67, name or relative path=path "Documents/FRC/DashboardSettings.ini") -> (appended path=w66:path)
  n175 = Build Path(base path=w67, name or relative path=path "Documents/FRC/Checklist.txt") -> (appended path=w71:path)
  n176 = call <vilib>:"Open Config Data.vi"("configuration file path"=w66) -> ("refnum"=w65:T25)  [unwired: 8 in, 2 out]
  n177 = call-poly <vilib>:"Read Key.vi"("section"=w62, "default value"="320x240", "key"="Size", "refnum"=w65) -> ("value"=w52:string, "refnum out"=w47:T25)  [unwired: 2 in, 4 out]
  n178 = Read from Text File(file (use dialog)=w71, count=-1 ("timeout ms (25000)")) -> (refnum out=w49:refnum<file>, text=w72:string[], error out=w73:errorcluster)  [unwired: 2 in, 1 out]
  n179 = case shown="No Error" w73 {
    tunnel: w72 -> [w311 _]
    tunnel: [w311 w313] -> w69
    tunnel: w70 -> [_ w313]
    tunnel: w71 -> [_ w314]
    tunnel: [w310 w312] -> w48
    tunnel: w49 -> [w310 _]
    frame No Error {
    }
    frame Error {
      n180 = Write to Text File(file (use dialog)=w314, text=w313) -> (refnum out=w312:refnum<file>)  [unwired: 2 in, 2 out]
    }
  }
  n181 = call-poly <vilib>:"Read Key.vi"("section"=w62, "default value"=30, "key"="FrameRate", "refnum"=w47) -> ("value"=w57:i32, "refnum out"=w46:T25)  [unwired: 1 in, 5 out]
  n182 = control-ref of="Tree"() -> (w43:refnum<vi>)
  n183 = property on="Listbox" class="LstBox (strict)"("Item Symbols"=i32[] [], "Item Names"=w69) -> ()  [unwired: 2 in, 2 out]
  n184 = Close File(refnum=w48) -> ()  [unwired: 1 in, 2 out]
  n185 = call-poly <vilib>:"Read Key.vi"("section"=w62, "default value"=30, "key"="Compression", "refnum"=w46) -> ("value"=w56:i32, "refnum out"=w44:T25)  [unwired: 1 in, 5 out]
  n186 = while {
    tunnel: [w316] -> _
    tunnel: w43 -> [w315]
    i -> [w316]
    stop <- FALSE stop-if-true
    n187 = Wait (ms)(milliseconds to wait=u32 60) -> ()  [unwired: 1 out]
    n188 = case shown="\"Variables\"" "Viewer" {
      tunnel: w315 -> [_ w320]
      frame Default {
      }
      frame "Variables" {
        n189 = call <vilib>:"NT Read and Format Entries as Tree.vi"("Tree Refnum"=w320) -> ()  [unwired: 9 in, 2 out]
      }
    }
  }
  n190 = control-ref of="Test Tree"() -> (w42:refnum<vi>)
  n191 = while {
    tunnel: w54 -> [w325]
    shift-right: [w324] -> _
    shift-left: w44 -> [w323]
    tunnel: [w322] -> _
    tunnel: w42 -> [w321]
    i -> [w322]
    stop <- FALSE stop-if-true
    n192 = event shown="[0] Timeout" {
      selector: _ -> [_ _ _ _ _ _ _ _ _ _ _ _ _]
      dyn-events: _ -> [_ _ _ _ _ _ _ _ _ _ _ _ _]
      timeout: u32 60 ("milliseconds to wait") -> [_ _ _ _ _ _ _ _ _ _ _ _ _]
      tunnel: w321 -> [w335 _ _ _ _ _ _ _ _ _ _ _ _]
      tunnel: "Test Tree" -> [_ _ _ _ _ _ _ _ w529 w537 w539 w543 w551]
      tunnel: w325 -> [_ w357 _ _ _ _ w493 w523 _ _ _ _ _]
      tunnel: [w329 w356 _ w459 w467 w479 w492 w516 w528 w535 w538 w542 w550] -> w324
      tunnel: w323 -> [w329 w356 _ w459 w467 w479 w491 w516 w528 w535 w538 w542 w550]
      event Timeout {
        w334 = enum16{"Update", "Clear"}[] [enum."Clear", enum."Clear", enum."Clear", enum."Clear", enum."Update", enum."Update", enum."Clear"] items=["Update", "Clear"]
        n193 = event-data() -> ()  [unwired: 1 in, 1 out]
        n194 = local read "Mode"() -> (w332:T6)
        n195 = Index Array(array=w334, index=w332) -> (element=w333:enum16{"Update", "Clear"})
        n196 = call <vilib>:"NT Read String.vi"("Name"="TestMode/TestName") -> ("String"=w338:string)  [unwired: 9 in, 1 out]
        n197 = case shown="\"Operation\", Default" "Dashboard Tab" {
          tunnel: w335 -> [_ w348]
          tunnel: "/TestMode/Automatic/" ("Name Pattern") -> [_ w347]
          tunnel: w333 -> [_ w346]
          tunnel: w332 -> [_ w344]
          frame "Operation", Default {
          }
          frame "Test" {
            w343 = -2 ("Active Item:Row Number")
            n198 = call <vilib>:"NT Read and Format Entries as Tree.vi"("Operation"=w346, "Name Pattern"=w347, "Tree Refnum"=w348) -> ()  [unwired: 7 in, 2 out]
            n199 = Index Array(array=u32[] [14013909, 14013909, 14013909, 14013909, 14013909, 16777215, 14013909], index=w344) -> (element=w342:u32)
            n200 = property on="Test Tree" class="Tree (strict)"("Active Item Row Number"=w343, "ActiveColNum"=w343, "CellBG"=w342, "Active Item Row Number"=-1 ("Active Item:Row Number"), "CellBG"=u32 5789784 ("Color Box")) -> ()  [unwired: 2 in, 2 out]
          }
        }
        n201 = case shown="\"\"" w338 {
          tunnel: "TestMode/TestProgress" ("Name") -> [w350 _]
          tunnel: "TestMode/TestProgressText" ("Name") -> [w349 _]
          frame Default {
            n202 = call <vilib>:"NT Read Number.vi"("Name"=w350) -> ("Numeric"=w351:dbl)  [unwired: 9 in, 1 out]
            n203 = call <vilib>:"NT Read String.vi"("Name"=w349) -> ("String"=w352:string)  [unwired: 9 in, 1 out]
            n204 = Bundle("Numeric"=w351, "String"=w352) -> (→"Progress":cluster{"Numeric":dbl, "String":string})  [unwired: 1 in]
          }
          frame "" {
            n205 = property on="Progress" class="Clust (strict)"("Visible"=FALSE) -> ()  [unwired: 2 in, 2 out]
            n206 = local write "Test Name"(u16 0) -> ()
          }
        }
      }
      event "Test Tree": Value Change {
        # "Show appropriate\ncontrols"
        n207 = event-data() -> ("CtlRef"=w360:refnum<vi>, "NewVal"=w358:string)  [unwired: 1 in]
        n208 = call <vilib>:"WPI_UtilitiesGetTreeIOName.vi"("NewVal"=w358, "TreeControl in"=w360) -> ("I/O Name"=w361:string)  [unwired: 9 in]
        n209 = case shown="\"Camera\"" w361 {
          selector: w361 -> [_ w368 _ w386 w395 _]
          tunnel: w358 -> [_ _ w383 w385 _ w402]
          tunnel: w357 -> [_ _ _ _ _ w401]
          frame Default {
            w363 = FALSE ("Visible")
            w362 = FALSE ("Visible")
            n210 = property on="Motor" class="Clust (strict)"("Visible"=w362) -> ()  [unwired: 2 in, 2 out]
            n211 = property on="Ring" class="Ring (strict)"("Visible"=w362) -> ()  [unwired: 2 in, 2 out]
            n212 = property on="Rev/Fwd" class="Clust (strict)"("Visible"=w363) -> ()  [unwired: 2 in, 2 out]
            n213 = property on="On/Off" class="Bool (strict)"("Visible"=w363) -> ()  [unwired: 2 in, 2 out]
            n214 = property on="Slider" class="Slide (strict)"("Visible"=w363) -> ()  [unwired: 2 in, 2 out]
          }
          frame "Motor", "PWM" {
            w369 = FALSE ("Visible")
            n215 = case shown="\"Motor\", Default" w368 {
              tunnel: [1.0 ("Value") -1.0 ("Value")] -> w367
              tunnel: [255.0 ("Value") 1.0 ("Value")] -> w366
              tunnel: [128.0 ("Value") 0.0 ("Value")] -> w365
              tunnel: [64.0 ("Value") 0.5 ("Value")] -> w364
              frame "PWM" {
              }
              frame "Motor", Default {
              }
            }
            n216 = property on="Motor" class="Clust (strict)"("Visible"=TRUE) -> ()  [unwired: 2 in, 2 out]
            n217 = property on="Value" class="Slide (strict)"("Value"=w365, "Scale.Minimum"=w367, "Scale.Maximum"=w366, "Scale.Increment"=w364) -> ()  [unwired: 2 in, 2 out]
            n218 = property on="On/Off" class="Bool (strict)"("Visible"=w369) -> ()  [unwired: 2 in, 2 out]
            n219 = property on="Slider" class="Slide (strict)"("Visible"=w369) -> ()  [unwired: 2 in, 2 out]
            n220 = property on="Ring" class="Ring (strict)"("Visible"=w369) -> ()  [unwired: 2 in, 2 out]
            n221 = property on="Rev/Fwd" class="Clust (strict)"("Visible"=w369) -> ()  [unwired: 2 in, 2 out]
          }
          frame "Servo" {
            w381 = FALSE ("Visible")
            n222 = call <vilib>:"NT Read Number.vi"("Name"=w383) -> ("Numeric"=w382:dbl)  [unwired: 9 in, 1 out]
            n223 = property on="Slider" class="Slide (strict)"("Visible"=TRUE, "Scale.Maximum"=170.0 ("Scale.Range:Maximum")) -> ()  [unwired: 2 in, 2 out]
            n224 = local write "Slider"(w382) -> ()
            n225 = property on="Motor" class="Clust (strict)"("Visible"=w381) -> ()  [unwired: 2 in, 2 out]
            n226 = property on="Rev/Fwd" class="Clust (strict)"("Visible"=w381) -> ()  [unwired: 2 in, 2 out]
            n227 = property on="On/Off" class="Bool (strict)"("Visible"=w381) -> ()  [unwired: 2 in, 2 out]
            n228 = property on="Ring" class="Ring (strict)"("Visible"=w381) -> ()  [unwired: 2 in, 2 out]
          }
          frame "Relay", "Solenoid" {
            w384 = FALSE ("Visible")
            n229 = property on="Motor" class="Clust (strict)"("Visible"=w384) -> ()  [unwired: 2 in, 2 out]
            n230 = property on="Slider" class="Slide (strict)"("Visible"=w384) -> ()  [unwired: 2 in, 2 out]
            n231 = Search and Replace String(input string=w385, search string="/Value  **", replace string="/Direction") -> (result string=w391:string)  [unwired: 5 in, 3 out]
            n232 = property on="Ring" class="Ring (strict)"("Visible"=w384) -> ()  [unwired: 2 in, 2 out]
            n233 = call <vilib>:"NT Read String.vi"("Name"=w391) -> ("String"=w389:string)  [unwired: 9 in, 1 out]
            n234 = Equal?(x="Both directions", y=w389) -> (x = y?=w387:bool)
            n235 = Not(x=w387) -> (.not. x?=w388:bool)
            n236 = property on="Rev/Fwd" class="Clust (strict)"("Visible"=w387) -> ()  [unwired: 2 in, 2 out]
            n237 = property on="On/Off" class="Bool (strict)"("Visible"=w388, "Caption.Text"=w386) -> ()  [unwired: 2 in, 2 out]
          }
          frame "Compressor", "Digital Out" {
            w394 = FALSE ("Visible")
            # "Get direction and finish"
            n238 = property on="Motor" class="Clust (strict)"("Visible"=w394) -> ()  [unwired: 2 in, 2 out]
            n239 = property on="Slider" class="Slide (strict)"("Visible"=w394) -> ()  [unwired: 2 in, 2 out]
            n240 = property on="Ring" class="Ring (strict)"("Visible"=w394) -> ()  [unwired: 2 in, 2 out]
            n241 = property on="On/Off" class="Bool (strict)"("Visible"=TRUE, "Caption.Text"=w395) -> ()  [unwired: 2 in, 2 out]
            n242 = property on="Rev/Fwd" class="Clust (strict)"("Visible"=FALSE) -> ()  [unwired: 2 in, 2 out]
          }
          frame "Camera" {
            n243 = call <vilib>:"Get Last Path Segment.vi"("String in"=w402) -> ("String out"=w403:string)  [unwired: 10 in]
            n244 = property on="On/Off" class="Bool (strict)"("Visible"=FALSE) -> ()  [unwired: 2 in, 2 out]
            n245 = property on="Motor" class="Clust (strict)"("Visible"=FALSE) -> ()  [unwired: 2 in, 2 out]
            n246 = property on="Rev/Fwd" class="Clust (strict)"("Visible"=FALSE) -> ()  [unwired: 2 in, 2 out]
            n247 = case shown="\"White Balance  **\"" w403 {
              tunnel: w402 -> [w409 w418 w427 w436 w445 _ w451]
              tunnel: w401 -> [w407 w415 w424 w433 w442 _ _]
              frame "Size  **" {
                n248 = Index Array(array=w407) -> (element=w406:cluster{string[]})  [unwired: 1 in]
                n249 = call <vilib>:"NT Read String.vi"("Name"=w409) -> ("String"=w408:string)  [unwired: 9 in, 1 out]
                n250 = Unbundle(w406) -> (w404:string[])
                n251 = Match First String(2:w404, 3:w408) -> (0:w405:i32)  [unwired: 1 out]
                n252 = property on="Ring" class="Ring (strict)"("Value"=w405, "Strings []"=w404) -> ()  [unwired: 2 in, 2 out]
                n253 = property on="Ring" class="Ring (strict)"("Visible"=TRUE) -> ()  [unwired: 2 in, 2 out]
                n254 = property on="Slider" class="Slide (strict)"("Visible"=FALSE) -> ()  [unwired: 2 in, 2 out]
              }
              frame "White Balance  **" {
                n255 = Index Array(array=w415, index=1) -> (element=w416:cluster{string[]})
                n256 = call <vilib>:"NT Read String.vi"("Name"=w418) -> ("String"=w417:string)  [unwired: 9 in, 1 out]
                n257 = Unbundle(w416) -> (w413:string[])
                n258 = Match First String(2:w413, 3:w417) -> (0:w412:i32)  [unwired: 1 out]
                n259 = property on="Ring" class="Ring (strict)"("Value"=w412, "Strings []"=w413) -> ()  [unwired: 2 in, 2 out]
                n260 = property on="Ring" class="Ring (strict)"("Visible"=TRUE) -> ()  [unwired: 2 in, 2 out]
                n261 = property on="Slider" class="Slide (strict)"("Visible"=FALSE) -> ()  [unwired: 2 in, 2 out]
              }
              frame "Exposure  **" {
                n262 = Index Array(array=w424, index=2) -> (element=w425:cluster{string[]})
                n263 = call <vilib>:"NT Read String.vi"("Name"=w427) -> ("String"=w426:string)  [unwired: 9 in, 1 out]
                n264 = Unbundle(w425) -> (w421:string[])
                n265 = Match First String(2:w421, 3:w426) -> (0:w422:i32)  [unwired: 1 out]
                n266 = property on="Ring" class="Ring (strict)"("Value"=w422, "Strings []"=w421) -> ()  [unwired: 2 in, 2 out]
                n267 = property on="Ring" class="Ring (strict)"("Visible"=TRUE) -> ()  [unwired: 2 in, 2 out]
                n268 = property on="Slider" class="Slide (strict)"("Visible"=FALSE) -> ()  [unwired: 2 in, 2 out]
              }
              frame "Exposure Priority  **" {
                n269 = Index Array(array=w433, index=3) -> (element=w434:cluster{string[]})
                n270 = call <vilib>:"NT Read String.vi"("Name"=w436) -> ("String"=w435:string)  [unwired: 9 in, 1 out]
                n271 = Unbundle(w434) -> (w430:string[])
                n272 = Match First String(2:w430, 3:w435) -> (0:w431:i32)  [unwired: 1 out]
                n273 = property on="Ring" class="Ring (strict)"("Value"=w431, "Strings []"=w430) -> ()  [unwired: 2 in, 2 out]
                n274 = property on="Ring" class="Ring (strict)"("Visible"=TRUE) -> ()  [unwired: 2 in, 2 out]
                n275 = property on="Slider" class="Slide (strict)"("Visible"=FALSE) -> ()  [unwired: 2 in, 2 out]
              }
              frame "Color Enable  **" {
                n276 = Index Array(array=w442, index=4) -> (element=w443:cluster{string[]})
                n277 = call <vilib>:"NT Read String.vi"("Name"=w445) -> ("String"=w444:string)  [unwired: 9 in, 1 out]
                n278 = Unbundle(w443) -> (w439:string[])
                n279 = Match First String(2:w439, 3:w444) -> (0:w440:i32)  [unwired: 1 out]
                n280 = property on="Ring" class="Ring (strict)"("Value"=w440, "Strings []"=w439) -> ()  [unwired: 2 in, 2 out]
                n281 = property on="Ring" class="Ring (strict)"("Visible"=TRUE) -> ()  [unwired: 2 in, 2 out]
                n282 = property on="Slider" class="Slide (strict)"("Visible"=FALSE) -> ()  [unwired: 2 in, 2 out]
              }
              frame Default {
                n283 = property on="Ring" class="Ring (strict)"("Visible"=FALSE) -> ()  [unwired: 2 in, 2 out]
                n284 = property on="Slider" class="Slide (strict)"("Visible"=FALSE) -> ()  [unwired: 2 in, 2 out]
              }
              frame "Brightness  **", "Color Level  **", "Compression  **", "FPS  **", "Sharpness  **" {
                n285 = call <vilib>:"NT Read Number.vi"("Name"=w451) -> ("Numeric"=w450:dbl)  [unwired: 9 in, 1 out]
                n286 = local write "Slider"(w450) -> ()
                n287 = property on="Slider" class="Slide (strict)"("Visible"=TRUE, "Scale.Maximum"=100.0 ("Scale.Range:Maximum")) -> ()  [unwired: 2 in, 2 out]
                n288 = property on="Ring" class="Ring (strict)"("Visible"=FALSE) -> ()  [unwired: 2 in, 2 out]
              }
            }
          }
        }
        n289 = property on="Progress" class="Clust (strict)"("Visible"=FALSE) -> ()  [unwired: 2 in, 2 out]
      }
      event "Test Name": Mouse Enter {
        # "Populate the ring with the list of tests"
        n290 = event-data() -> ()  [unwired: 1 in, 1 out]
        n291 = call <vilib>:"NT Read String Array.vi"("Name"="TestMode/TestList") -> ("String Array"=w458:string[])  [unwired: 9 in, 1 out]
        n292 = Build Array (concatenate)("Select the test to run...", w458) -> (w457:string[])
        n293 = property on="Test Name" class="Ring (strict)"("Strings []"=w457) -> ()  [unwired: 2 in, 2 out]
      }
      event "Test Name": Value Change {
        w460 = FALSE ("Visible")
        # "Tell the robot the test name to run"
        n294 = event-data() -> ("NewVal"=w464:u16)  [unwired: 1 in]
        n295 = property on="Test Name" class="Ring (strict)"() -> ("Strings []"=w465:string[])  [unwired: 2 in, 2 out]
        n296 = local write "Progress"(T7 {"Test Progress"=0, "Test Progress Text"=""} ("Progress")) -> ()
        n297 = Index Array(array=w465, index=w464) -> (element=w463:string)
        n298 = call <vilib>:"NT Write String.vi"("String"=w463, "Name"="TestMode/TestName") -> ()  [unwired: 9 in, 1 out]
        n299 = property on="Progress" class="Clust (strict)"("Visible"=TRUE) -> ()  [unwired: 2 in, 2 out]
        n300 = property on="Motor" class="Clust (strict)"("Visible"=w460) -> ()  [unwired: 2 in, 2 out]
        n301 = property on="Slider" class="Slide (strict)"("Visible"=w460) -> ()  [unwired: 2 in, 2 out]
        n302 = property on="On/Off" class="Bool (strict)"("Visible"=w460) -> ()  [unwired: 2 in, 2 out]
        n303 = property on="Rev/Fwd" class="Clust (strict)"("Visible"=w460) -> ()  [unwired: 2 in, 2 out]
        n304 = property on="Ring" class="Ring (strict)"("Visible"=w460) -> ()  [unwired: 2 in, 2 out]
      }
      event "Listbox": Double Click {
        n305 = event-data() -> ("PlatMods.Shift"=w468:bool, "Row"=w470:i32)  [unwired: 1 in]
        n306 = case shown="False" w468 {
          tunnel: w470 -> [w474 _]
          tunnel: 1 -> [w473 _]
          frame False {
            n307 = property on="Listbox" class="LstBox (strict)"() -> ("Item Symbols"=w472:i32[])  [unwired: 2 in, 2 out]
            n308 = Replace Array Subset(array=w472, new element=w473, index=w474) -> (w471:i32[])
            n309 = property on="Listbox" class="LstBox (strict)"("Item Symbols"=w471) -> ()  [unwired: 2 in, 2 out]
          }
          frame True {
            w475 = 0 ("Top Row")
            n310 = property on="Listbox" class="LstBox (strict)"() -> ("Number of Rows"=w477:u32)  [unwired: 2 in, 2 out]
            n311 = Initialize Array(0, w477) -> (w476:i32[])
            n312 = property on="Listbox" class="LstBox (strict)"("Top Row"=w475, "Value"=w475, "Item Symbols"=w476) -> ()  [unwired: 2 in, 2 out]
          }
        }
      }
      event "Listbox": Key Down {
        n313 = event-data() -> ("VKey"=w481:T26)  [unwired: 1 in]
        n314 = case shown="\"Left\", \"Right\"" w481 {
          selector: w481 -> [w486 _]
          tunnel: eventvkey."Left" ("VKey") -> [w484 _]
          frame "Left", "Right" {
            n315 = Equal?(x=w484, y=w486) -> (x = y?=w485:bool)
            n316 = Select(t=0, s=w485, f=1) -> (s? t:f=w487:i32)
            n317 = property on="Listbox" class="LstBox (strict)"() -> ("Item Symbols"=w490:i32[])  [unwired: 2 in, 2 out]
            n318 = Replace Array Subset(array=w490, new element=w487, index="Listbox") -> (w489:i32[])
            n319 = property on="Listbox" class="LstBox (strict)"("Item Symbols"=w489) -> ()  [unwired: 2 in, 2 out]
          }
          frame Default {
          }
        }
      }
      event "DB Camera Config": Value Change {
        n320 = event-data() -> ("NewVal"=w494:bool)  [unwired: 1 in]
        n321 = case shown="False" w494 {
          tunnel: w493 -> [w503 _]
          tunnel: [w496 w514] -> w492
          tunnel: w491 -> [w495 w514]
          frame False {
            w510 = "Camera"
            w513 = FALSE ("Visible")
            n322 = local read "Camera Settings"() -> (w502:T4)
            n323 = Index Array(array=w503) -> (element=w506:cluster{string[]})  [unwired: 1 in]
            n324 = Unbundle(w502) -> ("Frate Rate"=w501:i32, "Compression"=w500:i32, "Size"=w504:u16)
            n325 = Unbundle(w506) -> (w505:string[])
            n326 = Index Array(array=w505, index=w504) -> (element=w499:string)
            n327 = call-poly <vilib>:"Write Key.vi"("section"=w510, "value"=w499, "key"="Size", "refnum"=w495) -> ("refnum out"=w512:T25)  [unwired: 2 in, 5 out]
            n328 = call-poly <vilib>:"Write Key.vi"("section"=w510, "value"=w501, "key"="FrameRate", "refnum"=w512) -> ("refnum out"=w511:T25)  [unwired: 1 in, 6 out]
            n329 = property on="Camera Settings" class="Clust (strict)"("Visible"=w513) -> ()  [unwired: 2 in, 2 out]
            n330 = local write "DB Camera Config"(w513) -> ()
            n331 = call-poly <vilib>:"Write Key.vi"("section"=w510, "value"=w500, "key"="Compression", "refnum"=w511) -> ("refnum out"=w497:T25)  [unwired: 1 in, 6 out]
            n332 = call <vilib>:"Close Config Data.vi"("refnum"=w497) -> ("file path"=w498:path)  [unwired: 2 in, 8 out]
            n333 = call <vilib>:"Open Config Data.vi"("configuration file path"=w498) -> ("refnum"=w496:T25)  [unwired: 8 in, 2 out]
          }
          frame True {
            n334 = property on="Camera Settings" class="Clust (strict)"("Visible"=TRUE) -> ()  [unwired: 2 in, 2 out]
          }
        }
      }
      event "Camera Settings": Value Change {
        n335 = event-data() -> ("NewVal"=w527:T4)  [unwired: 1 in]
        n336 = Index Array(array=w523) -> (element=w522:cluster{string[]})  [unwired: 1 in]
        n337 = Unbundle(w527) -> ("Frate Rate"=w518:i32, "Compression"=w517:i32, "Size"=w520:u16)
        n338 = Unbundle(w522) -> (w521:string[])
        n339 = Index Array(array=w521, index=w520) -> (element=w519:string)
        n340 = Format Into String(format string="%s   %dfps   %d%%", w519, w518, w517) -> (resulting string=w524:string)  [unwired: 2 in, 1 out]
        n341 = Build Array(w524) -> (w525:string[])
        n342 = property on="DB Camera Config" class="Bool (strict)"("Strings [4]"=w525) -> ()  [unwired: 2 in, 2 out]
      }
      event "Motor.Enable": Value Change {
        n343 = event-data() -> ("NewVal"=w533:bool)  [unwired: 1 in]
        n344 = Unbundle("Motor") -> ("Value"=w532:dbl)  [unwired: 1 out]
        n345 = Select(t=w532, s=w533, f=0.0) -> (s? t:f=w530:dbl)
        n346 = call <vilib>:"NT Write Number.vi"("Numeric"=w530, "Name"=w529) -> ()  [unwired: 9 in, 1 out]
      }
      event "Slider": Value Change {
        n347 = event-data() -> ("NewVal"=w536:dbl)  [unwired: 1 in]
        n348 = call <vilib>:"NT Write Number.vi"("Numeric"=w536, "Name"=w537) -> ()  [unwired: 9 in, 1 out]
      }
      event "On/Off": Value Change {
        n349 = event-data() -> ("NewVal"=w541:bool)  [unwired: 1 in]
        n350 = Boolean To (0,1)(Boolean=w541) -> (0, 1=w540:i16)
        n351 = call <vilib>:"NT Write Number.vi"("Numeric"=w540, "Name"=w539) -> ()  [unwired: 9 in, 1 out]
      }
      event "Rev/Fwd": Value Change {
        n352 = event-data() -> ("NewVal.Forward"=w549:bool, "NewVal.Reverse"=w548:bool)  [unwired: 1 in]
        n353 = Boolean To (0,1)(Boolean=w549) -> (0, 1=w545:i16)
        n354 = Boolean To (0,1)(Boolean=w548) -> (0, 1=w547:i16)
        n355 = Negate(x=w547) -> (-x=w546:i16)
        n356 = Add(x=w545, y=w546) -> (x+y=w544:i16)
        n357 = call <vilib>:"NT Write Number.vi"("Numeric"=w544, "Name"=w543) -> ()  [unwired: 9 in, 1 out]
      }
      event "Ring": Value Change {
        n358 = event-data() -> ("NewVal"=w553:u16)  [unwired: 1 in]
        n359 = property on="Ring" class="Ring (strict)"() -> ("Strings []"=w554:string[])  [unwired: 2 in, 2 out]
        n360 = Index Array(array=w554, index=w553) -> (element=w552:string)
        n361 = call <vilib>:"NT Write String.vi"("String"=w552, "Name"=w551) -> ()  [unwired: 9 in, 1 out]
      }
    }
  }
  n362 = Index Array(array=w54) -> (element=w55:cluster{string[]})  [unwired: 1 in]
  n363 = Unbundle(w55) -> (w53:string[])
  n364 = Match First String(2:w53, 3:w52) -> (0:w51:i32)  [unwired: 1 out]
  n365 = Bundle("value"=w57, "value"=w56, "index"=w51) -> (w45:cluster{"value":i32, "value":i32, "index":i32})  [unwired: 1 out]
  n366 = property on="Camera Settings" class="Clust (strict)"("Val(Sgnl)"=w45) -> ()  [unwired: 2 in, 2 out]
  n367 = property on="On/Off" class="Bool (strict)"("Visible"=w68) -> ()  [unwired: 2 in, 2 out]
  n368 = property on="Motor" class="Clust (strict)"("Visible"=w68) -> ()  [unwired: 2 in, 2 out]
  n369 = property on="Progress" class="Clust (strict)"("Visible"=w68) -> ()  [unwired: 2 in, 2 out]
  n370 = property on="Ring" class="Ring (strict)"("Visible"=w68) -> ()  [unwired: 2 in, 2 out]
  n371 = property on="Rev/Fwd" class="Clust (strict)"("Visible"=w68) -> ()  [unwired: 2 in, 2 out]
  n372 = property on="Camera Settings" class="Clust (strict)"("Visible"=w68) -> ()  [unwired: 2 in, 2 out]
  n373 = local write "DB Camera Config"(w68) -> ()
  n374 = while {
    stop <- FALSE stop-if-true
    n375 = property on="Auto Align" class="Bool (strict)"() -> ("Value"=w563:bool)  [unwired: 2 in, 2 out]
    n376 = call "RisingEdgeDetect.vi"("Input"=w563) -> ("Output"=w562:bool)
    n377 = call "FallingEdgeDetect.vi"("Input"=w563) -> ("Output"=w559:bool)
    n378 = property on="Fine Control Mode" class="Bool (strict)"() -> ("Value"=w557:bool)  [unwired: 2 in, 2 out]
    n379 = Select(t=TRUE, s=w562, f=w557) -> (s? t:f=w558:bool)
    n380 = Select(t=FALSE, s=w559, f=w558) -> (s? t:f=w556:bool)
    n381 = property on="Fine Control Mode" class="Bool (strict)"("Val(Sgnl)"=w556) -> ()  [unwired: 2 in, 2 out]
  }
  n382 = while "Scanner Code" {
    i -> [w581]
    stop <- FALSE stop-if-true
    n383 = property on="Status" class="Enum (strict)"() -> ("Value"=w564:T2)  [unwired: 2 in, 2 out]
    n384 = Wait (ms)(milliseconds to wait=u32 300) -> ()  [unwired: 1 out]
    n385 = Quotient & Remainder(x=w581, y=6) -> (x-y*floor(x/y)=w583:i32)  [unwired: 1 out]
    n386 = case shown="\"Enabled\"" w564 {
      tunnel: [cluster{u32, u32}[] [{0, 0}, {0, 0}] ("Colors [4]") cluster{u32, u32}[] [{16711700, 16711700}, {16711700, 16711700}] ("Colors [4]") cluster{u32, u32}[] [{0, 16711700}, {16711700, 0}] ("Colors [4]") w589] -> w572
      frame "Disconnected" {
      }
      frame "E-Stop" {
      }
      frame "Disabled", Default {
      }
      frame "Enabled" {
        n387 = local read "Mode"() -> (w588:T6)
        n388 = case shown="\"Tele-Op Enabled\", Default" w588 {
          tunnel: [cluster{u32, u32}[] [{0, 1881090}, {1881090, 0}] ("Colors [4]") cluster{u32, u32}[] [{0, 11841800}, {11841800, 0}] ("Colors [4]") cluster{u32, u32}[] [{0, 983260}, {983260, 0}] ("Colors [4]")] -> w589
          frame "Tele-Op Enabled", Default {
          }
          frame "Auto Enabled" {
          }
          frame "Test Enabled" {
          }
        }
      }
    }
    n389 = case shown="0, Default" w583 {
      tunnel: [FALSE FALSE FALSE TRUE FALSE FALSE] -> w571
      tunnel: [FALSE FALSE TRUE FALSE TRUE FALSE] -> w570
      tunnel: [FALSE TRUE FALSE FALSE FALSE TRUE] -> w569
      tunnel: [TRUE FALSE FALSE FALSE FALSE FALSE] -> w568
      tunnel: [FALSE TRUE FALSE FALSE FALSE TRUE] -> w567
      tunnel: [FALSE FALSE TRUE FALSE TRUE FALSE] -> w566
      tunnel: [FALSE FALSE FALSE TRUE FALSE FALSE] -> w565
      frame 0, Default {
      }
      frame 1 {
      }
      frame 2 {
      }
      frame 3 {
      }
      frame 4 {
      }
      frame 5 {
      }
    }
    "Boolean" <- w571
    "Boolean 2" <- w570
    "Boolean 3" <- w569
    "Boolean 4" <- w568
    "Boolean 5" <- w567
    "Boolean 6" <- w566
    "Boolean 7" <- w565
    n390 = control-ref of="Boolean"() -> (w579:refnum<vi>)
    n391 = control-ref of="Boolean 2"() -> (w573:refnum<vi>)
    n392 = control-ref of="Boolean 3"() -> (w574:refnum<vi>)
    n393 = control-ref of="Boolean 4"() -> (w575:refnum<vi>)
    n394 = control-ref of="Boolean 5"() -> (w576:refnum<vi>)
    n395 = control-ref of="Boolean 6"() -> (w577:refnum<vi>)
    n396 = control-ref of="Boolean 7"() -> (w578:refnum<vi>)
    n397 = property class="Bool (strict)"(reference=w579, "Colors [4]"=w572) -> ()  [unwired: 1 in, 2 out]
    n398 = property class="Bool (strict)"(reference=w573, "Colors [4]"=w572) -> ()  [unwired: 1 in, 2 out]
    n399 = property class="Bool (strict)"(reference=w574, "Colors [4]"=w572) -> ()  [unwired: 1 in, 2 out]
    n400 = property class="Bool (strict)"(reference=w575, "Colors [4]"=w572) -> ()  [unwired: 1 in, 2 out]
    n401 = property class="Bool (strict)"(reference=w576, "Colors [4]"=w572) -> ()  [unwired: 1 in, 2 out]
    n402 = property class="Bool (strict)"(reference=w577, "Colors [4]"=w572) -> ()  [unwired: 1 in, 2 out]
    n403 = property class="Bool (strict)"(reference=w578, "Colors [4]"=w572) -> ()  [unwired: 1 in, 2 out]
  }
